vi "mks670_set_average.vi"() -> ()   [LabVIEW 2019]
panel:
  in  "averaging number":string
  out "Command Read":string
  out "tpg361_visa 3":refnum<visa-resource-name>
  out "err_out 2":errorcluster
  out "Status":bool
  in  "tpg361_b2r":u32
  in  "err_in":errorcluster
  in  "tpg361_delay":u32=500
  in  "tpg361_visa":refnum<visa-resource-name>
  # "VISA"
  # "DELAY"
  # "BYTE AT PORT"
  # "AVERAGE (1-100)"
  # "ERROR"
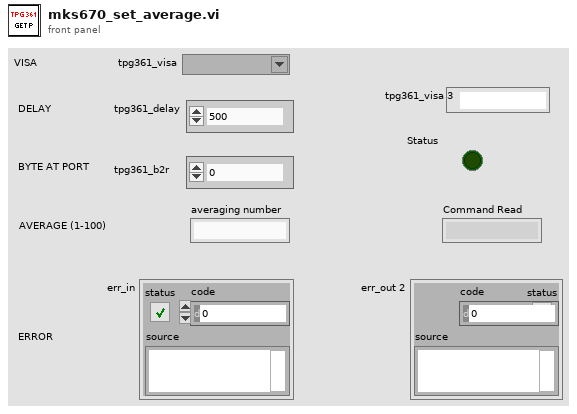
[diagram p1: front panel]
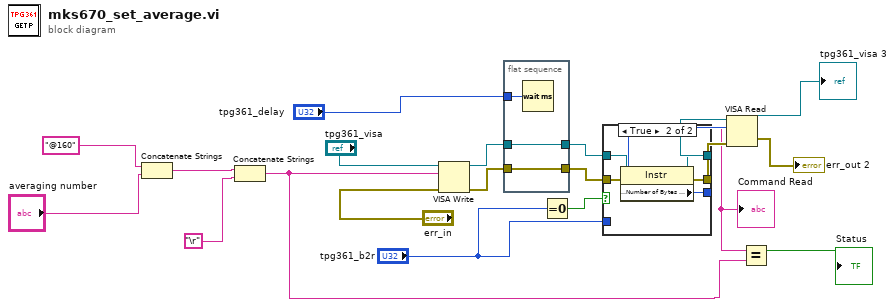
[diagram p0: block diagram]
diagram:
  n1 = Concatenate Strings("@160" ("string"), "averaging number") -> (w4:string)
  n2 = Concatenate Strings(w4, "\r") -> (w3:string)
  n3 = VISA Write(VISA resource name="tpg361_visa", write buffer=w3, error in (no error)="err_in") -> (VISA resource name out=w19:refnum<visa-resource-name>, error out=w21:errorcluster)  [unwired: 1 out]
  n4 = flat-sequence {
    tunnel: w21 -> [w23]
    tunnel: [w23] -> w20
    tunnel: w19 -> [w22]
    tunnel: [w22] -> w18
    tunnel: "tpg361_delay" -> [w24]
    frame #0 {
      n5 = Wait (ms)(milliseconds to wait=w24) -> ()  [unwired: 1 out]
    }
  }
  n6 = Equal To 0?(x="tpg361_b2r") -> (x = 0?=w14:bool)
  n7 = case shown="True" w14 {
    tunnel: w20 -> [w26 w32]
    tunnel: w18 -> [w27 w31]
    tunnel: [w27 w30] -> w12
    tunnel: [w26 w29] -> w11
    tunnel: [w25 w28] -> w10
    tunnel: "tpg361_b2r" -> [w25 _]
    frame False {
    }
    frame True {
      n8 = property class="Instr"(reference=w31, error in=w32) -> (reference out=w30:refnum<visa-resource-name>, error out=w29:errorcluster, "Serial Settings:Number of Bytes at Serial Port"=w28:u32)
    }
  }
  n9 = VISA Read(VISA resource name=w12, byte count=w10, error in (no error)=w11) -> (VISA resource name out=→"tpg361_visa 3":refnum<visa-resource-name>, read buffer=w8:string, error out=→"err_out 2":errorcluster)  [unwired: 1 out]
  "Command Read" <- w8
  n10 = Equal?(x=w8, y=w3) -> (x = y?=→"Status":bool)
